vi "Configure Reference Waveform.vi"   [LabVIEW 2017, in "Agilent 2000 3000 X-Series.lvlib"]
doc: "Configures reference waveform."
uses:
  Agilent 2000 3000 X-Series.lvlib
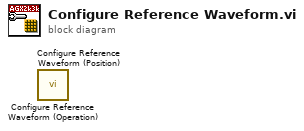
[diagram p0: block diagram]
diagram:
  n1 = call "Configure Reference Waveform (Operation).vi"() -> ()  [unwired: 10 in, 2 out]
  n2 = call "Configure Reference Waveform (Position).vi"() -> ()  [unwired: 10 in, 2 out]
